vi "Transport.CallByReference.vi"(8 "error in (no error)":errorcluster, 10 "method":T1=enum."LockinTimeDelay", 11 "Transport":refnum<class "Transport.lvclass">) -> (0 "error out":errorcluster)   [LabVIEW 2019, in "Transport.lvclass"]
uses:
  Transport.lvclass
  Typedefs/Transport.Methods--Enum.ctl
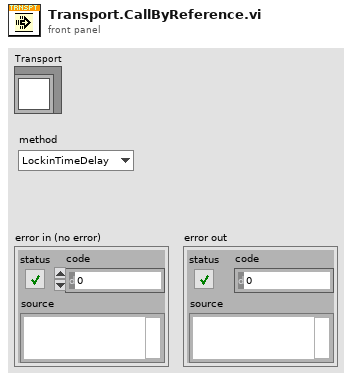
[diagram p1: front panel]
types:
  T1 = typedef "Transport.lvclass/Transport.Methods--Enum.ctl" = enum16{"LockinSweep", "LockinTime", "LockinTimeDelay"}
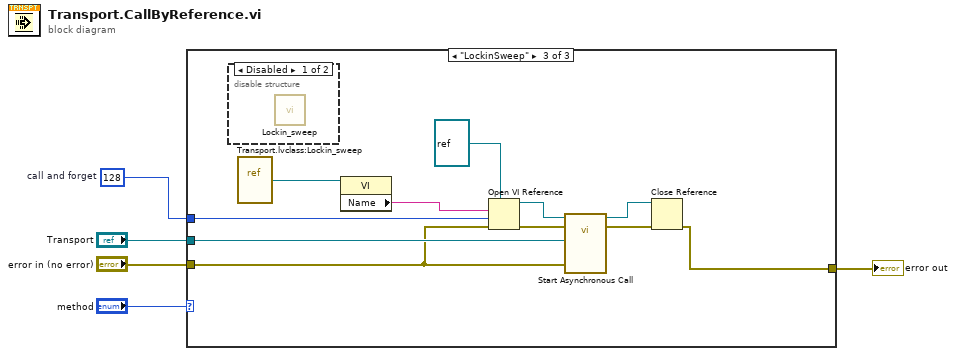
[diagram p0: block diagram]
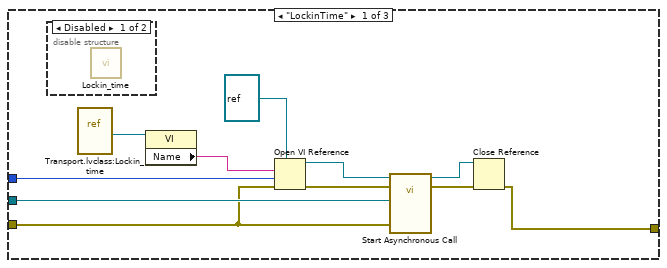
[diagram p2: hidden frame]
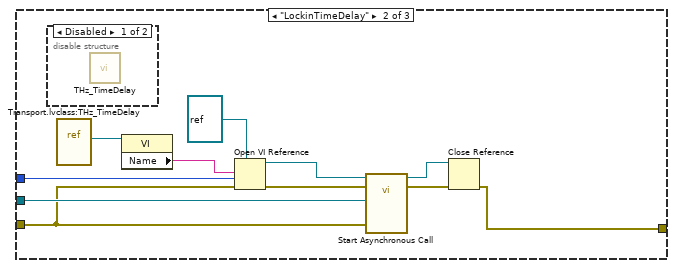
[diagram p4: hidden frame]
diagram:
  w1 = 128  # call and forget
  n1 = case shown="\"LockinSweep\"" "method" {
    tunnel: "Transport" -> [w15 w24 w38]
    tunnel: [w12 w21 w34] -> w2
    tunnel: "error in (no error)" -> [w11 w20 w31]
    tunnel: w1 -> [w10 w19 w30]
    frame "LockinTime" {
      n2 = disable-structure shown="Disabled" {
        frame Disabled {
          n3 = call "Lockin_time.vi"() -> ()  [unwired: 10 in, 2 out]
        }
        frame Enabled {
        }
      }
      n4 = vi-ref "Transport.lvclass:Lockin_time.vi"() -> (w9:refnum<vi>)
      n5 = property class="VI"(reference=w9) -> ("Name"=w7:string)  [unwired: 1 in, 2 out]
      n6 = Open VI Reference(type specifier VI Refnum (for type only)=refnum<vi> refnum, vi path=w7, options=w10, error in (no error)=w11) -> (vi reference=w6:refnum<vi>, error out=w16:errorcluster)  [unwired: 2 in]
      n7 = call-by-ref "Start Asynchronous Call"(reference=w6, error in=w16, 8:"error in (no error)"=w11, "Transport"=w15) -> (reference out=w13:refnum<vi>, error out=w14:errorcluster)  [unwired: 8 in, 2 out]
      n8 = Close Reference(reference=w13, error in (no error)=w14) -> (error out=w12:errorcluster)
    }
    frame "LockinTimeDelay" {
      n9 = disable-structure shown="Disabled" {
        frame Disabled {
          n10 = call "THz_TimeDelay.vi"() -> ()  [unwired: 10 in, 2 out]
        }
        frame Enabled {
        }
      }
      n11 = vi-ref "Transport.lvclass:THz_TimeDelay.vi"() -> (w18:refnum<vi>)
      n12 = property class="VI"(reference=w18) -> ("Name"=w17:string)  [unwired: 1 in, 2 out]
      n13 = Open VI Reference(type specifier VI Refnum (for type only)=refnum<vi> refnum, vi path=w17, options=w19, error in (no error)=w20) -> (vi reference=w25:refnum<vi>, error out=w26:errorcluster)  [unwired: 2 in]
      n14 = call-by-ref "Start Asynchronous Call"(reference=w25, error in=w26, 8:"error in (no error)"=w20, "Transport"=w24) -> (reference out=w23:refnum<vi>, error out=w22:errorcluster)  [unwired: 8 in, 2 out]
      n15 = Close Reference(reference=w23, error in (no error)=w22) -> (error out=w21:errorcluster)
    }
    frame "LockinSweep" {
      n16 = disable-structure shown="Disabled" {
        frame Disabled {
          n17 = call "Lockin_sweep.vi"() -> ()  [unwired: 9 in, 2 out]
        }
        frame Enabled {
        }
      }
      n18 = vi-ref "Transport.lvclass:Lockin_sweep.vi"() -> (w29:refnum<vi>)
      n19 = property class="VI"(reference=w29) -> ("Name"=w28:string)  [unwired: 1 in, 2 out]
      n20 = Open VI Reference(type specifier VI Refnum (for type only)=refnum<vi> refnum, vi path=w28, options=w30, error in (no error)=w31) -> (vi reference=w37:refnum<vi>, error out=w33:errorcluster)  [unwired: 2 in]
      n21 = call-by-ref "Start Asynchronous Call"(reference=w37, error in=w33, "Transport"=w38, 3:"error in (no error)"=w31) -> (reference out=w35:refnum<vi>, error out=w32:errorcluster)  [unwired: 7 in, 2 out]
      n22 = Close Reference(reference=w35, error in (no error)=w32) -> (error out=w34:errorcluster)
    }
  }
  "error out" <- w2
